vi "ReversedEngineering ConvertAttributesAndMethodsToString.vi"(1 "classInfo":T1, 5 "error in (no error)":errorcluster) -> (12 "StereoType":string, 15 "className":string, 16 "attributes":string, 17 "methods":string, 18 "ClassPath":path, 19 "error out":errorcluster)   [LabVIEW 2012]
uses:
  <resource>/Framework/Providers/Open_GDS/UML/ReversedEngineering/ReversedEngineering ClassInfoType.ctl
  <resource>/Framework/Providers/Open_GDS/UML/UMLEditor/UMLEditor_VisibilityType.ctl
  <resource>/Framework/Providers/Open_GDS/UML/ReversedEngineering/ReversedEngineering AttributeInfoType.ctl
  <resource>/Framework/Providers/Open_GDS/ClassProviders/Common/CommonVIs/CommonVIs_AttributeDataType.ctl
  <resource>/Framework/Providers/Open_GDS/UML/ReversedEngineering/ReversedEngineering_ClassDependencyDetailsType.ctl
  <resource>/Framework/Providers/Open_GDS/ClassProviders/Common/ScriptingFunctions/SubVIs/Scripting_ViDependencyType.ctl
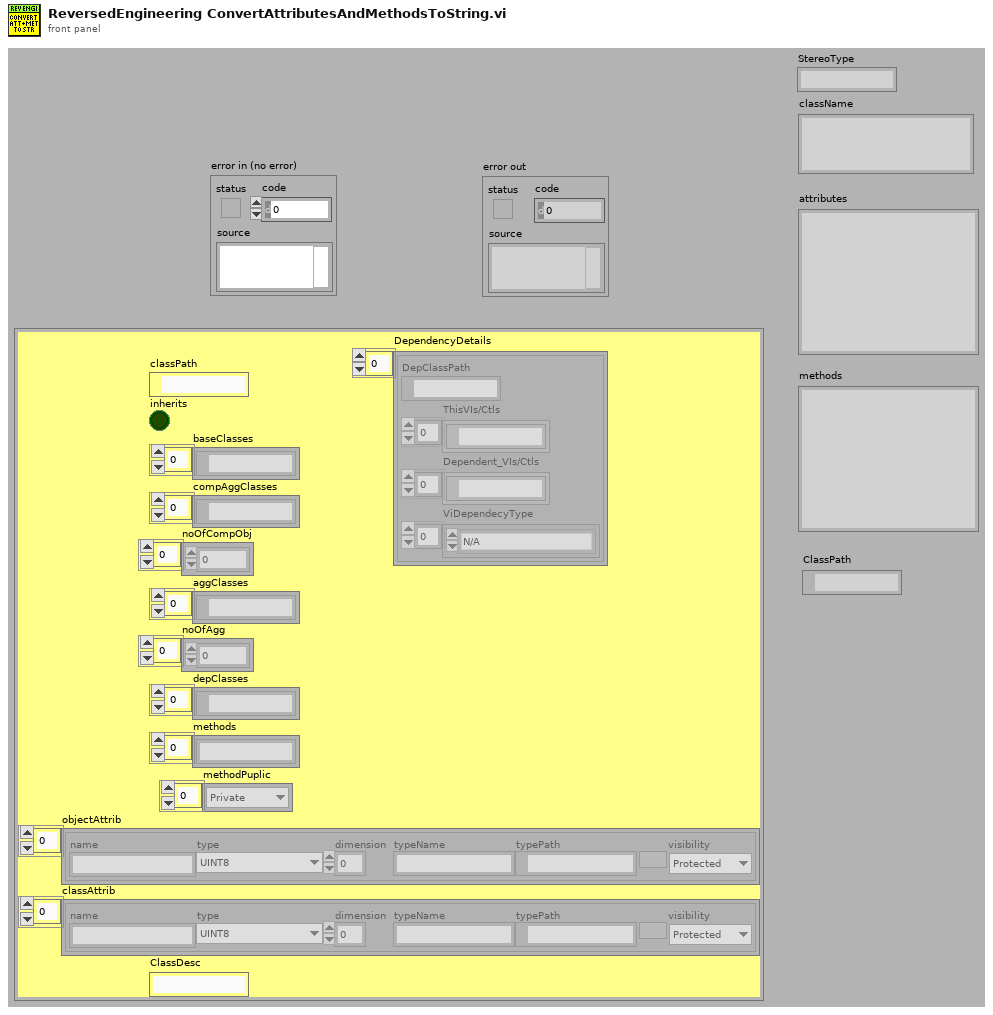
[diagram p1: front panel]
types:
  T1 = typedef "ReversedEngineering ClassInfoType.ctl" = cluster{"classPath":path, "inherits":bool, "baseClasses":path[], "compAggClasses":path[], "noOfCompObj":i32[], "aggClasses":path[], "noOfAgg":i32[], "depClasses":path[], "methods":string[], "methodPuplic":T2[], "objectAttrib":T3[], "classAttrib":T3[], "ClassDesc":string, "DependencyDetails":T5[]}
  T2 = typedef "UMLEditor_VisibilityType.ctl" = enum16{"Public", "Private", "Protected"}
  T3 = typedef "ReversedEngineering AttributeInfoType.ctl" = cluster{"name":string, "type":T4, "dimension":i32, "typeName":string, "typePath":path, "visibility":T2}
  T4 = typedef "CommonVIs_AttributeDataType.ctl" = enum16{"UINT8", "INT8", "UINT16", "INT16", "UINT32", "INT32", "UINT64", "INT64", "SGL", "DBL", "EXT", "CSG", "CDB", "CXT", "TimeStamp", "STRING", "PATH", "BOOL", "ENUM", "RefNum", "VIRefNum", "LabVIEW Class", "Cluster", "Variant", "TypeDef", "Waveform", "LabVIEW Object", "Other"}
  T5 = typedef "ReversedEngineering_ClassDependencyDetailsType.ctl" = cluster{"DepClassPath":path, "ThisVIs/Ctls":path[], "Dependent_VIs/Ctls":path[], "ViDependecyType":T6[]}
  T6 = typedef "Scripting_ViDependencyType.ctl" = enum16{"N/A", "Launches"}
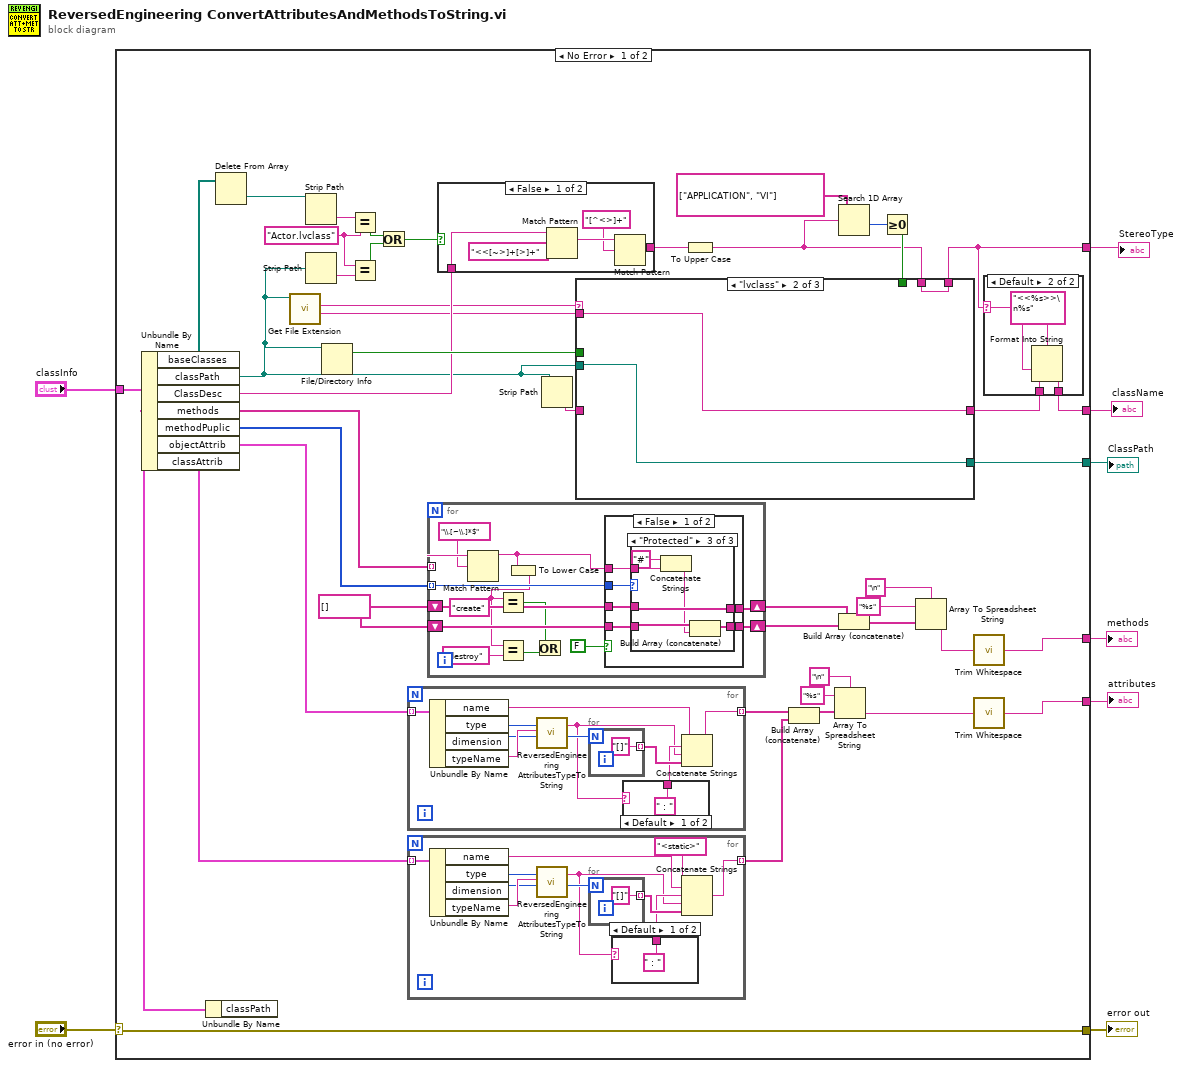
[diagram p0: block diagram]
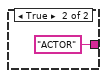
[diagram p2: hidden frame]
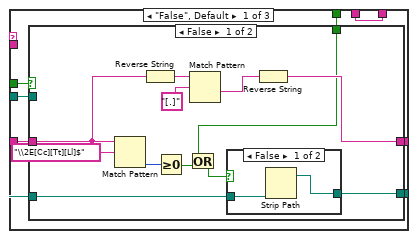
[diagram p3: hidden frame]
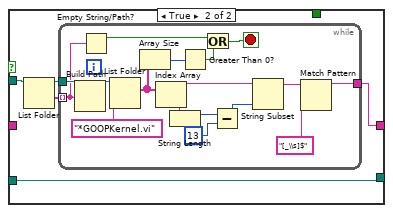
[diagram p5: hidden frame]
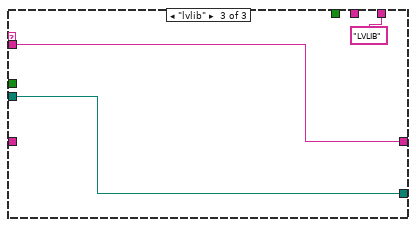
[diagram p6: hidden frame]
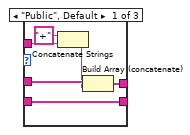
[diagram p10: hidden frame]
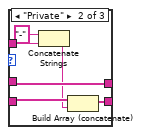
[diagram p11: hidden frame]
diagram:
  n1 = case shown="No Error" "error in (no error)" {
    selector: "error in (no error)" -> [w52 w176]
    tunnel: [w52 w176] -> w8
    tunnel: "classInfo" -> [w30 _]
    tunnel: [w26 _] -> w5
    tunnel: [w41 _] -> w4
    tunnel: [w32 _] -> w3
    tunnel: [w29 _] -> w2
    tunnel: [w19 _] -> w1
    frame No Error {
      w14 = "Actor.lvclass" ("y")
      w48 = string[] []
      n2 = Unbundle By Name(w30) -> ("baseClasses"=w17:path[], "classPath"=w10:path, "ClassDesc"=w28:string, "methods"=w49:string[], "methodPuplic"=w50:T2[], "objectAttrib"=w40:T3[], "classAttrib"=w39:T3[])
      n3 = Unbundle By Name(w30) -> ()  [unwired: 1 out]
      n4 = Delete From Array(array=w17) -> (deleted portion=w16:path)  [unwired: 2 in, 1 out]
      n5 = call <vilib>:"Get File Extension.vi"("file"=w10) -> ("filename without extension"=w22:string, "lowercase file extension"=w21:string)  [unwired: 1 in, 8 out]
      n6 = Strip Path(path=w16) -> (name=w18:string)  [unwired: 1 out]
      n7 = Strip Path(path=w10) -> (name=w15:string)  [unwired: 1 out]
      n8 = File/Directory Info(path=w10) -> (directory=w31:bool)  [unwired: 1 in, 6 out]
      n9 = Equal?(x=w18, y=w14) -> (x = y?=w12:bool)
      n10 = Equal?(x=w14, y=w15) -> (x = y?=w13:bool)
      n11 = Or(x=w12, y=w13) -> (x .or. y?=w11:bool)
      n12 = for {
        tunnel: w40 -> [w133] mode=indexing
        tunnel: [w128] -> w38 mode=indexing
        n13 = Unbundle By Name(w133) -> ("name"=w129:string, "type"=w132:T4, "dimension"=w130:i32, "typeName"=w131:string)
        n14 = call <resource>:"ReversedEngineering AttributesTypeToString.vi"("AttributeDataType"=w132, "name"=w131) -> ("string"=w125:string)  [unwired: 17 out]
        n15 = for {
          N: w130 -> [_]
          tunnel: ["[]"] -> w127 mode=indexing
        }
        n16 = case shown="Default" w125 {
          tunnel: [" : " _] -> w126
          frame Default {
          }
          frame "" {
          }
        }
        n17 = Concatenate Strings(w129, w126, w125, w127) -> (w128:string)
      }
      n18 = for {
        tunnel: w39 -> [w122] mode=indexing
        tunnel: [w117] -> w37 mode=indexing
        n19 = Unbundle By Name(w122) -> ("name"=w118:string, "type"=w121:T4, "dimension"=w119:i32, "typeName"=w120:string)
        n20 = call <resource>:"ReversedEngineering AttributesTypeToString.vi"("AttributeDataType"=w121, "name"=w120) -> ("string"=w113:string)  [unwired: 17 out]
        n21 = for {
          N: w119 -> [_]
          tunnel: ["[]"] -> w115 mode=indexing
        }
        n22 = case shown="Default" w113 {
          tunnel: [" : " _] -> w114
          frame Default {
          }
          frame "" {
          }
        }
        n23 = Concatenate Strings("<static>" ("string"), w118, w114, w113, w115) -> (w117:string)
      }
      n24 = for {
        tunnel: w50 -> [w149] mode=indexing
        tunnel: w49 -> [w140] mode=indexing
        shift-right: [w147] -> w47
        shift-left: w48 -> [w148]
        shift-right: [w145] -> w46
        shift-left: w48 -> [w146]
        n25 = Match Pattern(string=w140, regular expression="\\.[~\\.]*$") -> (before substring=w139:string)  [unwired: 4 out]
        n26 = To Lower Case(string=w139) -> (all lower case string=w138:string)
        n27 = Equal?(x=w138, y="create") -> (x = y?=w141:bool)
        n28 = Equal?(x=w138, y="destroy") -> (x = y?=w142:bool)
        n29 = Or(x=w141, y=w142) -> ()  [unwired: 1 out]
        n30 = case shown="False" FALSE {
          tunnel: w149 -> [w155 _]
          tunnel: w148 -> [w154 w175]
          tunnel: [w153 w175] -> w147
          tunnel: w146 -> [w152 w174]
          tunnel: [w151 w174] -> w145
          tunnel: w139 -> [w150 _]
          frame False {
            n31 = case shown="\"Protected\"" w155 {
              tunnel: w154 -> [w161 w167 w173]
              tunnel: [w160 w167 w173] -> w153
              tunnel: w152 -> [w159 w166 w172]
              tunnel: [w159 w165 w171] -> w151
              tunnel: w150 -> [w158 w164 w170]
              frame "Public", Default {
                n32 = Concatenate Strings("+" ("string"), w158) -> (w156:string)
                n33 = Build Array (concatenate)(w161, w156) -> (w160:string[])
              }
              frame "Private" {
                n34 = Concatenate Strings("-" ("string"), w164) -> (w162:string)
                n35 = Build Array (concatenate)(w166, w162) -> (w165:string[])
              }
              frame "Protected" {
                n36 = Concatenate Strings("#" ("string"), w170) -> (w168:string)
                n37 = Build Array (concatenate)(w172, w168) -> (w171:string[])
              }
            }
          }
          frame True {
          }
        }
      }
      n38 = case shown="False" w11 {
        tunnel: w28 -> [w54 _]
        tunnel: [w53 "ACTOR" ("ClassDesc")] -> w20
        frame False {
          n39 = Match Pattern(string=w54, regular expression="<<[~>]+[>]+") -> (match substring=w57:string)  [unwired: 4 out]
          n40 = Match Pattern(string=w57, regular expression="[^<>]+") -> (match substring=w53:string)  [unwired: 4 out]
        }
        frame True {
        }
      }
      n41 = Strip Path(path=w10) -> (name=w51:string)  [unwired: 1 out]
      n42 = To Upper Case(1:w20) -> (0:w9:string)
      n43 = Build Array (concatenate)(w38, w37) -> (w34:string[])
      n44 = Array To Spreadsheet String(delimiter (Tab)="\n", array=w34, 3:"%s" ("format string")) -> (spreadsheet string=w33:string)
      n45 = Search 1D Array(1D array=string[] ["APPLICATION", "VI"], element=w9) -> (index of element=w24:i32)  [unwired: 1 out]
      n46 = Build Array (concatenate)(w47, w46) -> (w45:string[])
      n47 = Greater Or Equal To 0?(x=w24) -> (x >= 0?=w23:bool)
      n48 = case shown="\"lvclass\"" w21 {
        tunnel: w51 -> [w65 _ _]
        tunnel: w31 -> [w64 _ _]
        tunnel: [w63 w103 w105] -> w29
        tunnel: [w62 w104 w106] -> w27
        tunnel: w23 -> [w61 _ _]
        tunnel: w10 -> [w60 w103 w105]
        tunnel: w22 -> [_ w104 w106]
        tunnel: w9 -> [w59 w102 _]
        tunnel: [w59 w102 "LVLIB" ("ClassDesc")] -> w19
        frame "False", Default {
          n49 = case shown="False" w64 {
            tunnel: w65 -> [w71 _]
            tunnel: [w72 w85] -> w62
            tunnel: w60 -> [_ w84]
            tunnel: [w73 w81] -> w63
            tunnel: w60 -> [w74 w81]
            tunnel: w61 -> [w67 _]
            frame False {
              n50 = Match Pattern(string=w71, regular expression="\\2E[Cc][Tt][Ll]$") -> (offset past match=w69:i32)  [unwired: 4 out]
              n51 = Reverse String(1:w71) -> (0:w77:string)
              n52 = Greater Or Equal To 0?(x=w69) -> (x >= 0?=w68:bool)
              n53 = Or(x=w67, y=w68) -> (x .or. y?=w66:bool)
              n54 = Match Pattern(string=w77, regular expression="[.]") -> (after substring=w75:string)  [unwired: 4 out]
              n55 = case shown="False" w66 {
                tunnel: w74 -> [w79 w80]
                tunnel: [w78 w80] -> w73
                frame False {
                  n56 = Strip Path(path=w79) -> (stripped path=w78:path)  [unwired: 1 out]
                }
                frame True {
                }
              }
              n57 = Reverse String(1:w75) -> (0:w72:string)
            }
            frame True {
              n58 = List Folder(path=w84) -> (path out=w83:path, folder names=w82:string[])  [unwired: 1 in, 4 out]
              n59 = while {
                tunnel: [w94] -> w85
                tunnel: w83 -> [w92]
                tunnel: w82 -> [w89] mode=indexing
                stop <- w86 stop-if-true
                n60 = Build Path(base path=w92, name or relative path=w89) -> (appended path=w91:path)
                n61 = Empty String/Path?(string/path=w89) -> (empty?=w88:bool)
                n62 = List Folder(path=w91, pattern="*GOOPKernel.vi") -> (filenames=w93:string[])  [unwired: 1 in, 4 out]
                n63 = Array Size(array=w93) -> (size(s)=w90:i32)
                n64 = Index Array(array=w93) -> (element=w100:string)  [unwired: 1 in]
                n65 = String Length(string=w100) -> (length=w99:i32)
                n66 = Greater Than 0?(x=w90) -> (x > 0?=w87:bool)
                n67 = Or(x=w88, y=w87) -> (x .or. y?=w86:bool)
                n68 = Subtract(x=w99, y=13) -> (x-y=w97:i32)
                n69 = String Subset(string=w100, length (rest)=w97) -> (substring=w96:string)  [unwired: 1 out]
                n70 = Match Pattern(string=w96, regular expression="[_\\s]$") -> (before substring=w94:string)  [unwired: 4 out]
              }
            }
          }
        }
        frame "lvclass" {
        }
        frame "lvlib" {
        }
      }
      n71 = Array To Spreadsheet String(delimiter (Tab)="\n", array=w45, 3:"%s" ("format string")) -> (spreadsheet string=w42:string)
      n72 = call <vilib>:"Trim Whitespace.vi"("string"=w42) -> ("trimmed string"=w41:string)  [unwired: 1 in]
      n73 = call <vilib>:"Trim Whitespace.vi"("string"=w33) -> ("trimmed string"=w32:string)  [unwired: 1 in]
      n74 = case shown="Default" w19 {
        selector: w19 -> [_ w112]
        tunnel: w27 -> [w108 w110]
        tunnel: [w108 w109] -> w26
        frame "" {
        }
        frame Default {
          n75 = Format Into String(format string="<<%s>>\n%s", w112, w110) -> (resulting string=w109:string)  [unwired: 2 in, 1 out]
        }
      }
    }
    frame Error {
    }
  }
  "error out" <- w8
  "attributes" <- w3
  "className" <- w5
  "methods" <- w4
  "ClassPath" <- w2
  "StereoType" <- w1
